vi "Analysis_Widefield.vi"(5 "Spatial filter size (um)":i32=5, 6 "error in (no error)":errorcluster, 8 "Image_odor":sgl[][](array[numeric]), 9 "Image_air":sgl[][](array[numeric])) -> (0 "error out":errorcluster, 3 "single precision float":sgl[][](array[numeric]))   [LabVIEW 2014]
uses:
  Widefield_globals.vi
  <vilib>/vision/NI_Vision_Development_Module.lvlib
panel:
  # "only write a header\nif repeat=1"
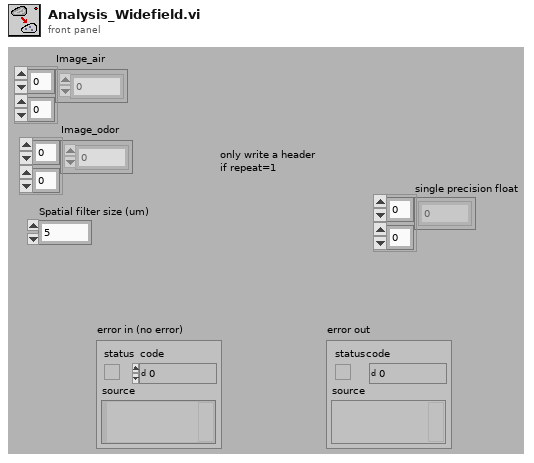
[diagram p1: front panel]
types:
  T1 = enum32{"", "Gradient", "Laplacian", "Smoothing", "Gaussian"}
  T2 = typedef "IMAQ Image.ctl" = refnum<image>
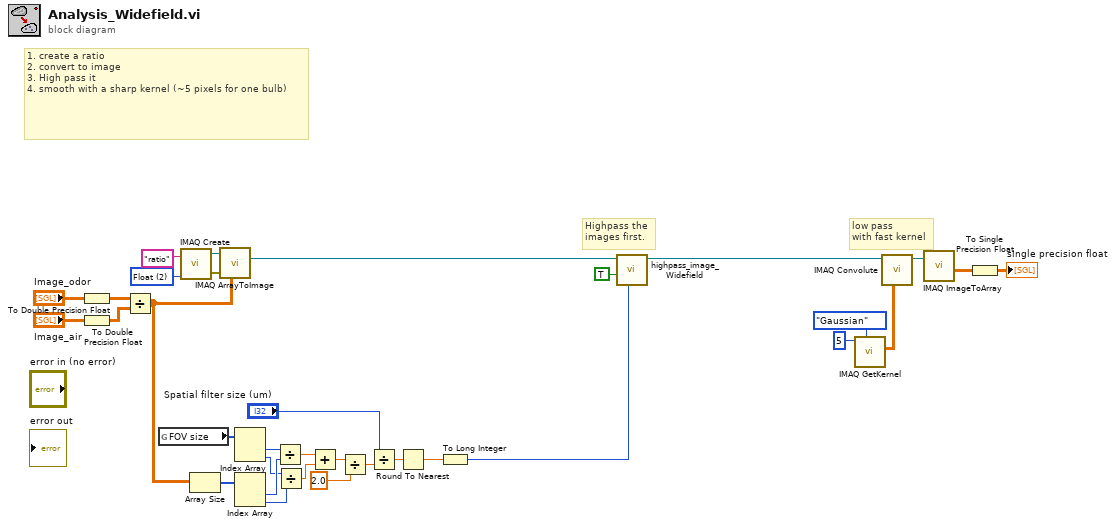
[diagram p0: block diagram]
diagram:
  w31 = u32 2 items=["8 bits", "16 bits", "Float", "Complex", "RGB", "HSL"] ("Image Type")
  # "Highpass the\nimages first."
  # "low pass\nwith fast kernel"
  # "1. create a ratio \n2. convert to image\n3. High pass it\n4. smooth with a sharp kernel (~5 pixels for one bulb)"
  n1 = To Double Precision Float(number="Image_odor") -> (double precision float=w28:dbl[][])
  n2 = To Double Precision Float(number="Image_air") -> (double precision float=w29:dbl[][])
  n3 = Divide(x=w28, y=w29) -> (x/y=w17:dbl[][])
  n4 = global read "Widefield_globals.vi" "FOV size"() -> (w15:i32[])
  n5 = call "IMAQ Create"("Image Name"="ratio", "Image Type"=w31) -> ("New Image"=w33:T2, "error out"=w32:errorcluster)  [unwired: 2 in, 1 out]
  n6 = Array Size(array=w17) -> (size(s)=w16:i32[])
  n7 = call "IMAQ ArrayToImage"("Image Pixels (Float)"=w17, "error in (no error)"=w32, "Image"=w33) -> ("Image Out"=w27:T2)  [unwired: 3 in, 5 out]
  n8 = Index Array(array=w15) -> (element #1=w14:i32, element #2=w12:i32)  [unwired: 2 in]
  n9 = Index Array(array=w16) -> (element #1=w13:i32, element #2=w11:i32)  [unwired: 2 in]
  n10 = Divide(x=w14, y=w13) -> (x/y=w10:dbl)
  n11 = Divide(x=w12, y=w11) -> (x/y=w9:dbl)
  n12 = Add(x=w10, y=w9) -> (x+y=w8:dbl)
  n13 = Divide(x=w8, y=2.0) -> (x/y=w6:dbl)
  n14 = Divide(x="Spatial filter size (um)", y=w6) -> (x/y=w4:dbl)
  n15 = Round To Nearest(number=w4) -> (nearest integer value=w3:dbl)
  n16 = To Long Integer(number=w3) -> (32bit integer=w2:i32)
  n17 = call "highpass_image_Widefield.vi"("Gauss size"=w2, "One Bulb?"=TRUE, "Image"=w27) -> ("high passed image"=w20:T2)  [unwired: 8 in]
  n18 = call "IMAQ GetKernel"("Kernel Family"=T1."Gaussian", "Kernel Size (3,5,...)"=5) -> ("Kernel"=w22:sgl[][])  [unwired: 3 in, 6 out]
  n19 = call "IMAQ Convolute"("Kernel"=w22, "Image Src"=w20) -> ("Image Dst Out"=w19:T2)  [unwired: 5 in, 4 out]
  n20 = call "IMAQ ImageToArray"("Image"=w19) -> ("Image Pixels (Float)"=w24:sgl[][])  [unwired: 2 in, 5 out]
  n21 = To Single Precision Float(number=w24) -> (single precision float=→"single precision float":sgl[][])
